vi "Thermo Gas Conc Read (SubVI).vi"(8 "Error In":errorcluster, 11 "Instrument":T3(ring)) -> (0 "error out":errorcluster, 3 "Data Out":T2(array[cluster]))   [LabVIEW 2010]
uses:
  Program Files/National Instruments/LabVIEW 2012/vi.lib/NI Modbus.llb/MB Ethernet Master Query Read Holding Registers (poly).vi
  <vilib>/Utility/error.llb/DialogType.ctl
panel:
  in  "?":T1(tab)
  in  "NOx IP":string="192.168.1.201"
  in  "Quantity NOx":u16=6
  in  "MBAP Header NOx":cluster{"Transaction ID":u16, "Unit ID":u8}={"Transaction ID"=0, "Unit ID"=42}
  in  "SO2 IP":string="192.168.1.202"
  in  "Quantity  SO2":u16=2
  in  "MBAP Header  SO2":cluster{"Transaction ID":u16, "Unit ID":u8}={"Transaction ID"=0, "Unit ID"=43}
  in  "O3 IP":string="192.168.1.203"
  in  "Quantity O3":u16=2
  in  "MBAP Header  O3":cluster{"Transaction ID":u16, "Unit ID":u8}={"Transaction ID"=0, "Unit ID"=49}
  in  "Starting Address":u16
  in  "remote port":u16=502
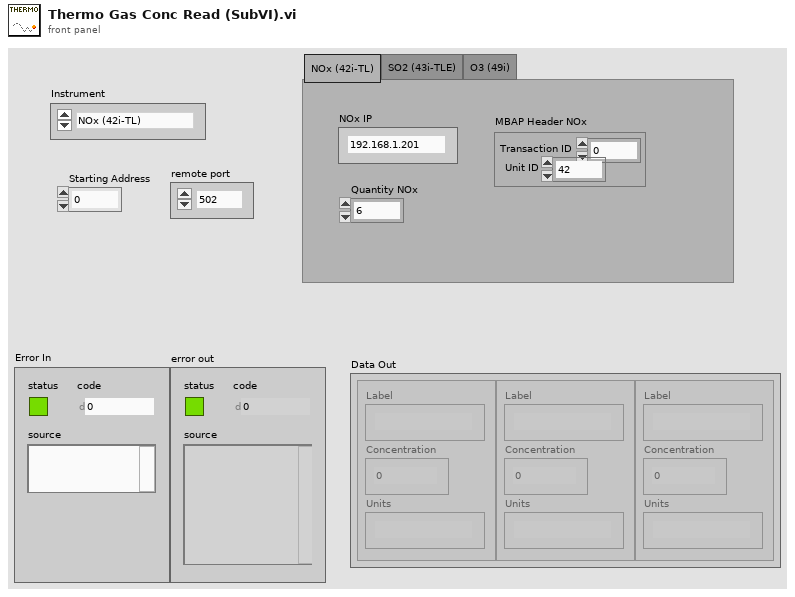
[diagram p1: front panel]
types:
  T1 = enum32{"NOx (42i-TL)", "SO2 (43i-TLE)", "O3 (49i)"}
  T2 = cluster{"Label":string, "Concentration":sgl, "Units":string}[]
  T3 = enum16{"NOx (42i-TL)", "SO2 (43i-TLE)", "O3 (49i)"}
  T4 = typedef "DialogType.ctl" = u16
  T5 = cluster{"Label":string, "Concentration":sgl, "Units":string}
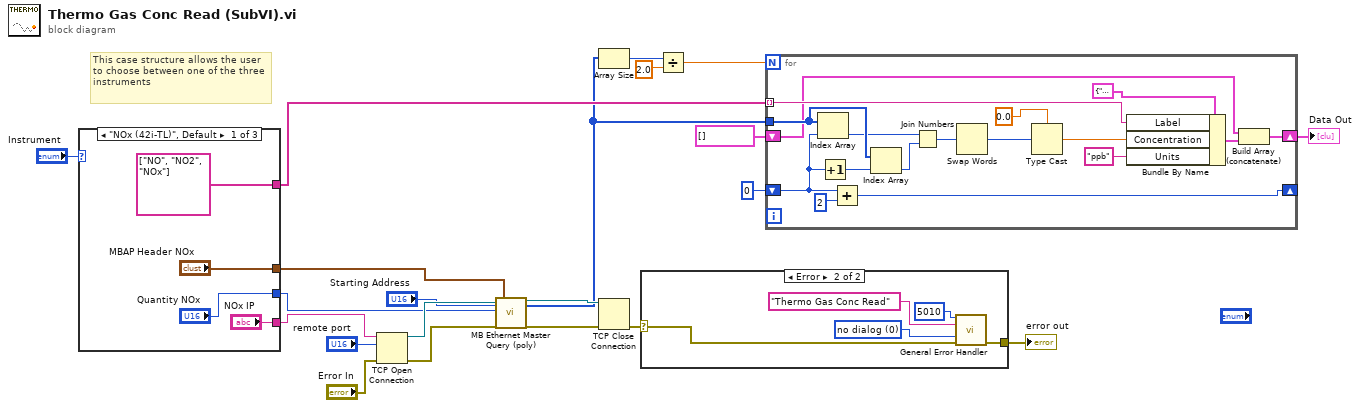
[diagram p0: block diagram]
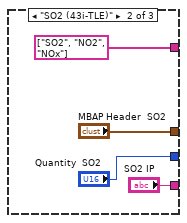
[diagram p3: hidden frame]
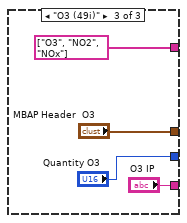
[diagram p4: hidden frame]
diagram:
  # "This case structure allows the user to choose between one of the three instruments"
  n1 = case shown="\"NOx (42i-TL)\", Default" "Instrument" {
    tunnel: ["MBAP Header NOx" "MBAP Header  SO2" "MBAP Header  O3"] -> w15
    tunnel: ["NOx IP" "SO2 IP" "O3 IP"] -> w14
    tunnel: ["Quantity NOx" "Quantity  SO2" "Quantity O3"] -> w13
    tunnel: [string[] ["NO", "NO2", "NOx"] string[] ["SO2", "NO2", "NOx"] string[] ["O3", "NO2", "NOx"]] -> w11
    frame "NOx (42i-TL)", Default {
    }
    frame "SO2 (43i-TLE)" {
    }
    frame "O3 (49i)" {
    }
  }
  n2 = TCP Open Connection(address=w14, remote port or service name="remote port", error in (no error)="Error In") -> (connection ID=w19:refnum<k5>, error out=w18:errorcluster)  [unwired: 2 in]
  n3 = call-poly "MB Ethernet Master Query (poly).vi"("TCP Connection Refnum in"=w19, "Starting Address"="Starting Address", "Quantity"=w13, "error in"=w18, "MBAP Header"=w15) -> ("TCP Connection Refnum (dup)"=w21:refnum<k5>, "Holding Registers"=w4:u16[], "error out"=w20:errorcluster)  [unwired: 11 in, 1 out]
  n4 = Array Size(array=w4) -> (size(s)=w9:i32)
  n5 = TCP Close Connection(connection ID=w21, error in (no error)=w20) -> (error out=w1:errorcluster)  [unwired: 1 in, 1 out]
  n6 = case shown="Error" w1 {
    selector: w1 -> [w34 w36]
    tunnel: [w34 w35] -> w2
    frame No Error {
    }
    frame Error {
      w37 = T4 0 items=["no dialog", "OK message", "continue or stop message", "OK message + warnings", "continue/stop + warnings"] ("type of dialog (OK msg:1)")
      n7 = call <vilib>:"General Error Handler.vi"("[error code] (0)"=5010, "[error source] (\" \")"="Thermo Gas Conc Read" ("[error source] (\" \")"), "type of dialog (OK msg:1)"=w37, "error in (no error)"=w36) -> ("error out"=w35:errorcluster)  [unwired: 7 in, 4 out]
    }
  }
  "error out" <- w2
  n8 = Divide(x=w9, y=2.0) -> (x/y=w8:dbl)
  n9 = for {
    N: w8 -> [_]
    tunnel: w4 -> [w56]
    tunnel: w11 -> [w48] mode=indexing
    shift-right: [w41] -> w5
    shift-left: T2 [] -> [w40]
    shift-right: [w47] -> _
    shift-left: 0 -> [w45]
    n10 = Index Array(array=w56, index=w45) -> (element=w53:u16)
    n11 = Increment(x=w45) -> (x+1=w44:i32)
    n12 = Add(x=w45, y=2) -> (x+y=w47:i32)
    n13 = Index Array(array=w56, index=w44) -> (element=w52:u16)
    n14 = Join Numbers(hi=w53, lo=w52) -> ((hi.lo)=w54:u32)
    n15 = Swap Words(1:w54) -> (0:w51:u32)
    n16 = Type Cast(type=sgl 0.0, x=w51) -> (*(type *) &x=w50:sgl)
    n17 = Bundle By Name(cluster=T5 {"Label"="", "Concentration"=0.0, "Units"=""}, "Label"=w48, "Concentration"=w50, "Units"="ppb") -> (w43:T5)
    n18 = Build Array (concatenate)(w40, w43) -> (w41:T2)
  }
  "Data Out" <- w5
